vi "SubVI_DataBuf.vi"(7 "cmd":enum16{"ini", "write", "read"}(ring), 8 "error in (no error)":errorcluster caption="에러 입력(에러 없음)", 11 "Total data":T1={"Raw Data"={"Res_data"=[], "Acc_data"={"t0"=timestamp(0 s since 1904-01-01), "dt"=1.0, "Y"=[]}, "Strain_data"=[]}, "Resister result data"={"Resistor values"={"[0]"=0.0, "[1]"=0.0, "[2]"=0.0, "[3]"=0.0, "[4]"=0.0, "[5]"=0.0, "[6]"=0.0, "[7]"=0.0, "[8]"=0.0, "[9]"=0.0, "[10]"=0.0, "[11]"=0.0, "[12]"=0.0, "[13]"=0.0, "[14]"=0.0}, "Resistor tables"=[], "Pass Fails"=[]}, "Result Table update"={"Num"=[], "Resister 1~5"=[], "Resister 6~10"=[], "Resister 11~15"=[]}, "Strain Data"={"Strain 1"=0.003117022901603048, "Strain 2"=0.003117022901603048, "Strain 3"=0.003117022901603048, "Strain 4"=0.003117022901603048}, "Acc Result"={"Acc Peak"=1.576875651161608, "Acc time"=0.00041000000000000005, "Acc area"=0.00033609583207321286}, "STATUS"={"status"="exit", "all_fail"=FALSE, "emg"=FALSE, "cycle"=10, "file name"=""}, "Speed"=0.0, "Acc peak time"=0.0, "Max Strain"=0.0, "Resistor at peak"={"[0]"=0.0, "[1]"=0.0, "[2]"=0.0, "[3]"=0.0, "[4]"=0.0, "[5]"=0.0, "[6]"=0.0, "[7]"=0.0, "[8]"=0.0, "[9]"=0.0, "[10]"=0.0, "[11]"=0.0, "[12]"=0.0, "[13]"=0.0, "[14]"=0.0}, "Acc peak index"=0, "time"="", "Cycle finish"=FALSE, "Resistor at ini"={"[0]"=0.0, "[1]"=0.0, "[2]"=0.0, "[3]"=0.0, "[4]"=0.0, "[5]"=0.0, "[6]"=0.0, "[7]"=0.0, "[8]"=0.0, "[9]"=0.0, "[10]"=0.0, "[11]"=0.0, "[12]"=0.0, "[13]"=0.0, "[14]"=0.0}} {"Strain Data"."Strain 4" format="%#.2f"; "Strain Data"."Strain 3" format="%#.2f"; "Strain Data"."Strain 2" format="%#.2f"; "Strain Data"."Strain 1" format="%#.2f"; "Acc Result"."Acc area" format="%#.2f"; "Acc Result"."Acc time" format="%#.2p"; "Acc Result"."Acc Peak" format="%#.2f"}) -> (0 "error out":errorcluster caption="에러 출력", 3 "Total data 2":T1={"Raw Data"={"Res_data"=[], "Acc_data"={"t0"=timestamp(0 s since 1904-01-01), "dt"=1.0, "Y"=[]}, "Strain_data"=[]}, "Resister result data"={"Resistor values"={"[0]"=0.0, "[1]"=0.0, "[2]"=0.0, "[3]"=0.0, "[4]"=0.0, "[5]"=0.0, "[6]"=0.0, "[7]"=0.0, "[8]"=0.0, "[9]"=0.0, "[10]"=0.0, "[11]"=0.0, "[12]"=0.0, "[13]"=0.0, "[14]"=0.0}, "Resistor tables"=[], "Pass Fails"=[]}, "Result Table update"={"Num"=[], "Resister 1~5"=[], "Resister 6~10"=[], "Resister 11~15"=[]}, "Strain Data"={"Strain 1"=0.003117022901603048, "Strain 2"=0.003117022901603048, "Strain 3"=0.003117022901603048, "Strain 4"=0.003117022901603048}, "Acc Result"={"Acc Peak"=1.576875651161608, "Acc time"=0.00041000000000000005, "Acc area"=0.00033609583207321286}, "STATUS"={"status"="exit", "all_fail"=FALSE, "emg"=FALSE, "cycle"=10, "file name"=""}, "Speed"=0.0, "Acc peak time"=0.0, "Max Strain"=0.0, "Resistor at peak"={"[0]"=0.0, "[1]"=0.0, "[2]"=0.0, "[3]"=0.0, "[4]"=0.0, "[5]"=0.0, "[6]"=0.0, "[7]"=0.0, "[8]"=0.0, "[9]"=0.0, "[10]"=0.0, "[11]"=0.0, "[12]"=0.0, "[13]"=0.0, "[14]"=0.0}, "Acc peak index"=0, "time"="", "Cycle finish"=FALSE, "Resistor at ini"={"[0]"=0.0, "[1]"=0.0, "[2]"=0.0, "[3]"=0.0, "[4]"=0.0, "[5]"=0.0, "[6]"=0.0, "[7]"=0.0, "[8]"=0.0, "[9]"=0.0, "[10]"=0.0, "[11]"=0.0, "[12]"=0.0, "[13]"=0.0, "[14]"=0.0}} {"Strain Data"."Strain 4" format="%#.2f"; "Strain Data"."Strain 3" format="%#.2f"; "Strain Data"."Strain 2" format="%#.2f"; "Strain Data"."Strain 1" format="%#.2f"; "Acc Result"."Acc area" format="%#.2f"; "Acc Result"."Acc time" format="%#.2p"; "Acc Result"."Acc Peak" format="%#.2f"})   [LabVIEW 2016]
uses:
  Ctrls/Total data.ctl
  Ctrls/raw Q data.ctl
  Ctrls/raw data type.ctl
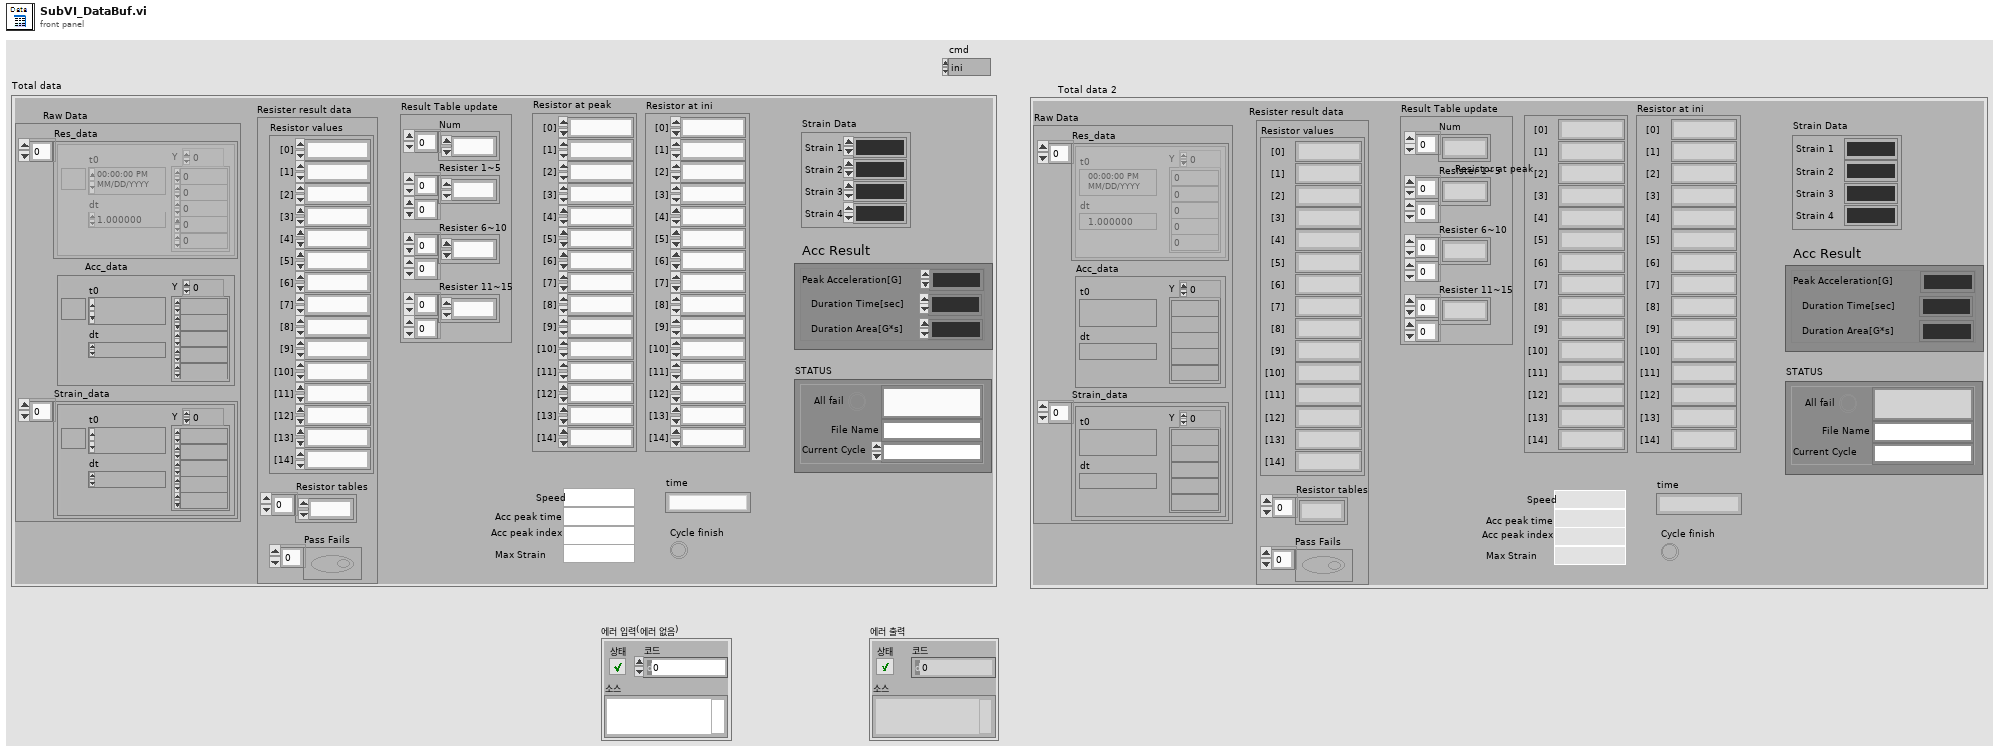
[diagram p1: front panel]
types:
  T1 = typedef "Total data.ctl" = cluster{"Raw Data":T2, "Resister result data":T3, "Result Table update":cluster{"Num":u32[], "Resister 1~5":u8[][], "Resister 6~10":u8[][], "Resister 11~15":u8[][]}, "Strain Data":cluster{"Strain 1":dbl, "Strain 2":dbl, "Strain 3":dbl, "Strain 4":dbl}, "Acc Result":cluster{"Acc Peak":dbl, "Acc time":dbl, "Acc area":dbl}, "STATUS":cluster{"status":string, "all_fail":bool, "emg":bool, "cycle":u16, "file name":string}, "Speed":dbl, "Acc peak time":dbl, "Max Strain":dbl, "Resistor at peak":cluster{"[0]":dbl, "[1]":dbl, "[2]":dbl, "[3]":dbl, "[4]":dbl, "[5]":dbl, "[6]":dbl, "[7]":dbl, "[8]":dbl, "[9]":dbl, "[10]":dbl, "[11]":dbl, "[12]":dbl, "[13]":dbl, "[14]":dbl}, "Acc peak index":u32, "time":string, "Cycle finish":bool, "Resistor at ini":cluster{"[0]":dbl, "[1]":dbl, "[2]":dbl, "[3]":dbl, "[4]":dbl, "[5]":dbl, "[6]":dbl, "[7]":dbl, "[8]":dbl, "[9]":dbl, "[10]":dbl, "[11]":dbl, "[12]":dbl, "[13]":dbl, "[14]":dbl}}
  T2 = typedef "raw Q data.ctl" = cluster{"Res_data":waveform(dbl)[], "Acc_data":waveform(dbl), "Strain_data":waveform(dbl)[]}
  T3 = typedef "raw data type.ctl" = cluster{"Resistor values":cluster{"[0]":dbl, "[1]":dbl, "[2]":dbl, "[3]":dbl, "[4]":dbl, "[5]":dbl, "[6]":dbl, "[7]":dbl, "[8]":dbl, "[9]":dbl, "[10]":dbl, "[11]":dbl, "[12]":dbl, "[13]":dbl, "[14]":dbl}, "Resistor tables":u8[], "Pass Fails":bool[]}
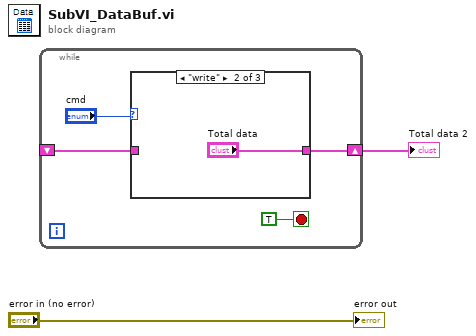
[diagram p0: block diagram]
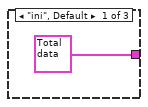
[diagram p2: hidden frame]
diagram:
  n1 = while {
    shift-right: [w4] -> w1
    shift-left: _ -> [w3]
    stop <- TRUE stop-if-true
    n2 = case shown="\"write\"" "cmd" {
      tunnel: [T1 {"Raw Data"={"Res_data"=[], "Acc_data"={"t0"=timestamp(0 s since 1904-01-01), "dt"=1.0, "Y"=[]}, "Strain_data"=[]}, "Resister result data"={"Resistor values"={"[0]"=0.0, "[1]"=0.0, "[2]"=0.0, "[3]"=0.0, "[4]"=0.0, "[5]"=0.0, "[6]"=0.0, "[7]"=0.0, "[8]"=0.0, "[9]"=0.0, "[10]"=0.0, "[11]"=0.0, "[12]"=0.0, "[13]"=0.0, "[14]"=0.0}, "Resistor tables"=[], "Pass Fails"=[]}, "Result Table update"={"Num"=[], "Resister 1~5"=[], "Resister 6~10"=[], "Resister 11~15"=[]}, "Strain Data"={"Strain 1"=0.0, "Strain 2"=0.0, "Strain 3"=0.0, "Strain 4"=0.0}, "Acc Result"={"Acc Peak"=0.0, "Acc time"=0.0, "Acc area"=0.0}, "STATUS"={"status"="", "all_fail"=FALSE, "emg"=FALSE, "cycle"=0, "file name"=""}, "Speed"=0.0, "Acc peak time"=0.0, "Max Strain"=0.0, "Resistor at peak"={"[0]"=0.0, "[1]"=0.0, "[2]"=0.0, "[3]"=0.0, "[4]"=0.0, "[5]"=0.0, "[6]"=0.0, "[7]"=0.0, "[8]"=0.0, "[9]"=0.0, "[10]"=0.0, "[11]"=0.0, "[12]"=0.0, "[13]"=0.0, "[14]"=0.0}, "Acc peak index"=0, "time"="", "Cycle finish"=FALSE, "Resistor at ini"={"[0]"=0.0, "[1]"=0.0, "[2]"=0.0, "[3]"=0.0, "[4]"=0.0, "[5]"=0.0, "[6]"=0.0, "[7]"=0.0, "[8]"=0.0, "[9]"=0.0, "[10]"=0.0, "[11]"=0.0, "[12]"=0.0, "[13]"=0.0, "[14]"=0.0}} ("Total data 2") "Total data" w9] -> w4
      tunnel: w3 -> [_ _ w9]
      frame "ini", Default {
      }
      frame "write" {
      }
      frame "read" {
      }
    }
  }
  "Total data 2" <- w1
  "error out" <- "error in (no error)"
